vi "Add Time Stamp.vi"(8 "error in (no error)":errorcluster, 11 "Running Log":string) -> (0 "error out":errorcluster, 3 "String":string)   [LabVIEW 2014, in "Testing UI 1.lvlib"]
uses:
  Testing UI 1.lvlib
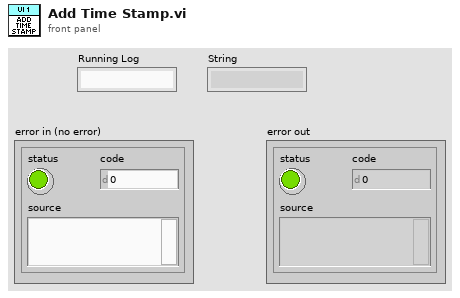
[diagram p1: front panel]
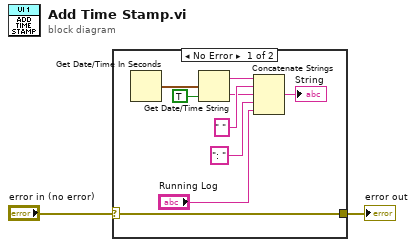
[diagram p0: block diagram]
diagram:
  n1 = case shown="No Error" "error in (no error)" {
    selector: "error in (no error)" -> [w3 w12]
    tunnel: [w3 w12] -> w1
    frame No Error {
      n2 = Get Date/Time In Seconds() -> (seconds since 1Jan1904=w5:timestamp)
      n3 = Get Date/Time String(seconds (now)=w5, want seconds? (F)=TRUE) -> (date string=w6:string, time string=w10:string)  [unwired: 1 in]
      n4 = Concatenate Strings(w6, " " ("string"), w10, ": " ("string"), "Running Log") -> (→"String":string)
    }
    frame Error {
    }
  }
  "error out" <- w1
